vi "Solve1.vi"(8 "Error In":errorcluster, 11 "object in":refnum<class "2021_10.lvclass">) -> (0 "Error Out":errorcluster, 2 "Result":u64, 3 "object out":refnum<class "2021_10.lvclass">)   [LabVIEW 2020, in "2021_10.lvclass"]
uses:
  2021_10.lvclass
panel:
  out "Corrupted Lines":cluster{i32, "string":string}[](array[cluster])
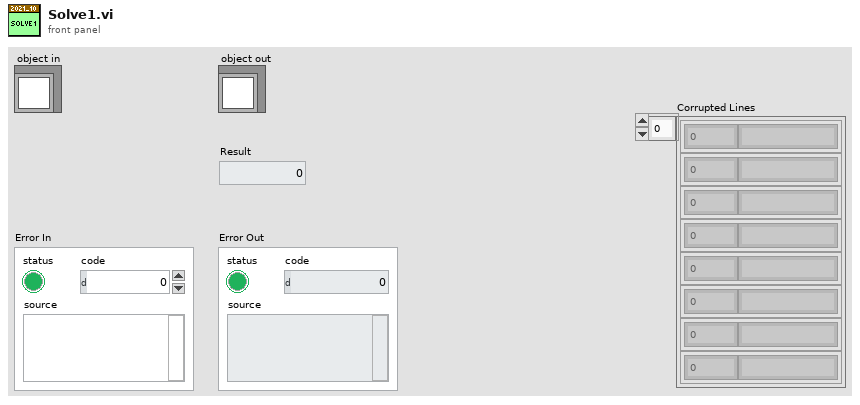
[diagram p1: front panel]
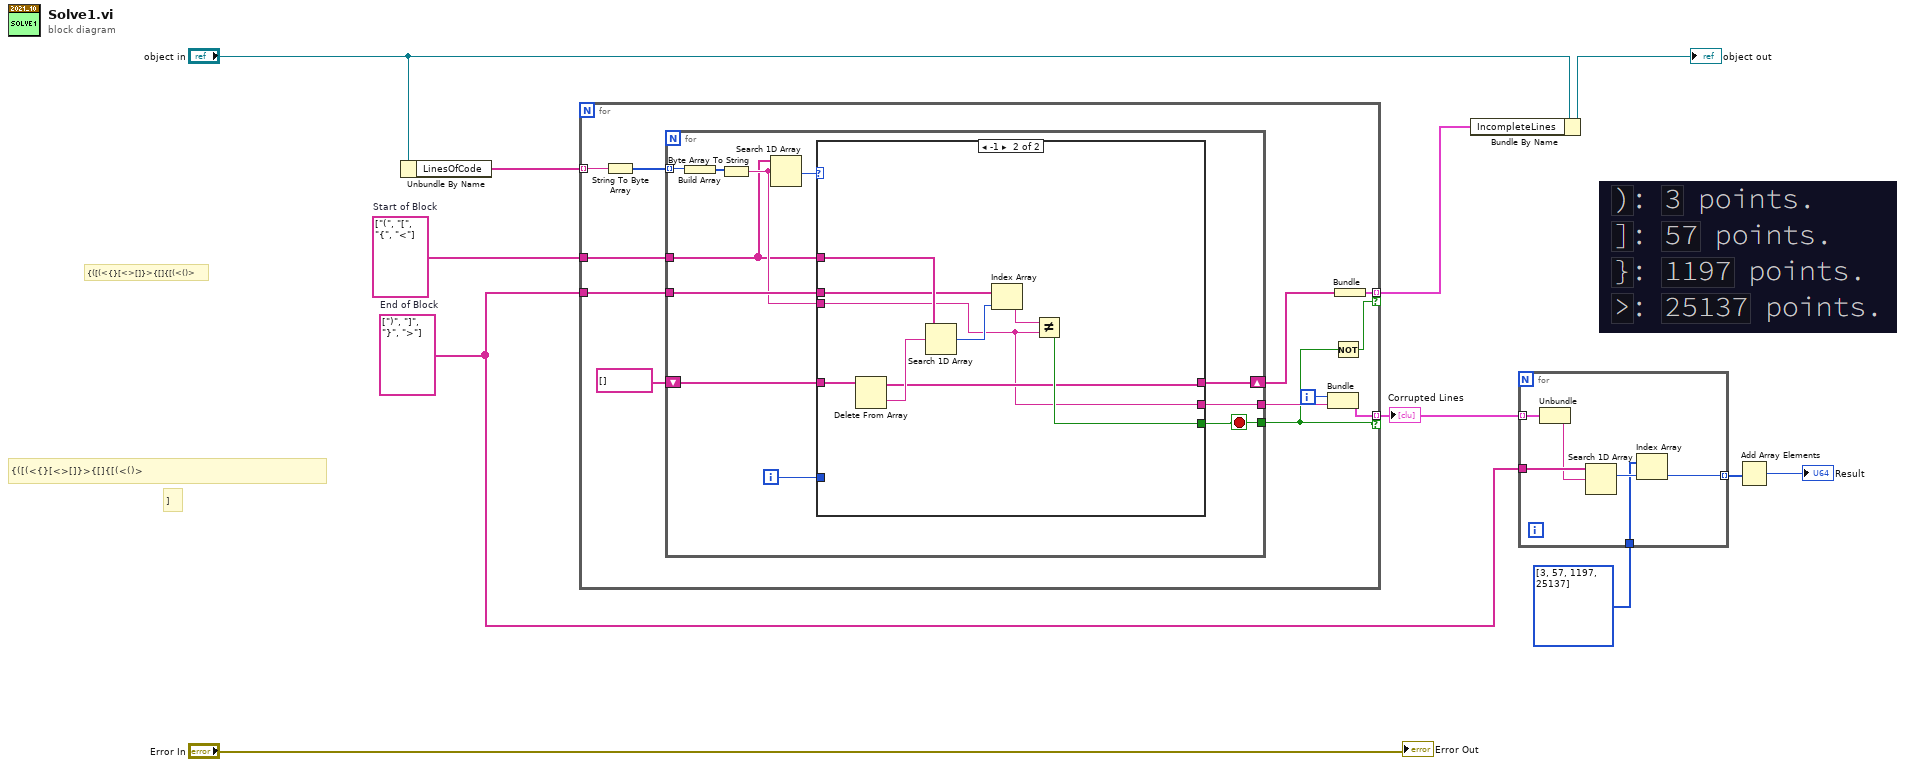
[diagram p0: block diagram]
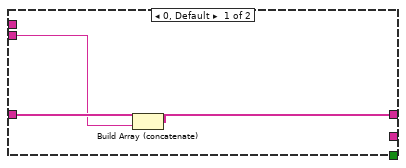
[diagram p2: hidden frame]
diagram:
  w6 = string[] [")", "]", "}", ">"]  # End of Block
  w8 = string[] ["(", "[", "{", "<"]  # Start of Block
  # "]"
  # "{([(<{}[<>[]}>{[]{[(<()>"
  # "{([(<{}[<>[]}>{[]{[(<()>"
  n1 = Unbundle By Name("object in") -> ("LinesOfCode"=w9:string[])
  n2 = for {
    tunnel: w9 -> [w15] mode=indexing
    tunnel: w8 -> [w22]
    tunnel: w6 -> [w21]
    tunnel: [w18] -> w7 mode=indexing if=w16
    tunnel: [w13] -> w1 mode=indexing if=w12
    i -> [w20]
    n3 = String To Byte Array(string=w15) -> (unsigned byte array=w23:u8[])
    n4 = for {
      tunnel: w23 -> [w34] mode=indexing
      tunnel: w22 -> [w25]
      shift-right: [w30] -> w14
      shift-left: string[] [] -> [w31]
      tunnel: w21 -> [w29]
      tunnel: [w27] -> w16
      tunnel: [w24] -> w19
      i -> [w26]
      stop <- w27 stop-if-true
      n5 = Build Array(w34) -> (w33:u8[])
      n6 = Byte Array To String(unsigned byte array=w33) -> (string=w28:string)
      n7 = Search 1D Array(1D array=w25, element=w28) -> (index of element=w32:i32)  [unwired: 1 in]
      n8 = case shown="-1" w32 {
        tunnel: w31 -> [w37 w46]
        tunnel: [w35 w39] -> w30
        tunnel: w29 -> [_ w43]
        tunnel: w28 -> [w36 w38]
        tunnel: [_ w40] -> w27
        tunnel: w26 -> [_ _]
        tunnel: w25 -> [_ w44]
        tunnel: [_ w38] -> w24
        frame 0, Default {
          n9 = Build Array (concatenate)(w37, w36) -> (w35:string[])
        }
        frame -1 {
          n10 = Delete From Array(array=w46) -> (deleted portion=w45:string, array with subset deleted=w39:string[])  [unwired: 2 in]
          n11 = Search 1D Array(1D array=w44, element=w45) -> (index of element=w42:i32)  [unwired: 1 in]
          n12 = Index Array(array=w43, index=w42) -> (element=w41:string)
          n13 = Not Equal?(x=w41, y=w38) -> (x != y?=w40:bool)
        }
      }
    }
    n14 = Bundle(w20, "string"=w19) -> (w18:cluster{i32, "string":string})  [unwired: 1 in]
    n15 = Not(x=w16) -> (.not. x?=w12:bool)
    n16 = Bundle(w14) -> (w13:cluster{string[]})  [unwired: 1 in]
  }
  "Corrupted Lines" <- w7
  n17 = Bundle By Name(cluster="object in", "IncompleteLines"=w1) -> (→"object out":refnum<class "2021_10.lvclass">)
  n18 = for {
    tunnel: w7 -> [w52] mode=indexing
    tunnel: w6 -> [w51]
    tunnel: u64[] [3, 57, 1197, 25137] -> [w48]
    tunnel: [w47] -> w4 mode=indexing
    n19 = Unbundle(w52) -> ("string"=w50:string)  [unwired: 1 out]
    n20 = Search 1D Array(1D array=w51, element=w50) -> (index of element=w49:i32)  [unwired: 1 in]
    n21 = Index Array(array=w48, index=w49) -> (element=w47:u64)
  }
  n22 = Add Array Elements(numeric array=w4) -> (sum=→"Result":u64)
  "Error Out" <- "Error In"
